vi "Handle State Value Table Change.vi"(8 "error in (no error)":errorcluster, 9 "OldVal":T1[](array[typedef]), 10 "NewVal":T1[](array[typedef]), 11 "routing channel in":T2 format="%.0x") -> (0 "error out":errorcluster, 1 "old modified state and value":T1, 2 "new modified state and value":T1, 3 "routing channel out":T2 format="%.0x", 4 "update controls":bool, 5 "coerced newval":T1[](array[typedef]))   [LabVIEW 2020, in "Routing and Faulting System Explorer.lvlib"]
uses:
  Routing and Faulting System Explorer.lvlib
  <vilib>/NI VeriStand/Custom Device API/Custom Device Item Ref.ctl
  State-Value Row.ctl
  88e8a73d-5bf6-438f-825b-ec6305f3fa8d.vi
  Scripting/Routing and Faulting Scripting.lvlib
  <vilib>/NI VeriStand/Custom Device API/Custom Device API.lvlib
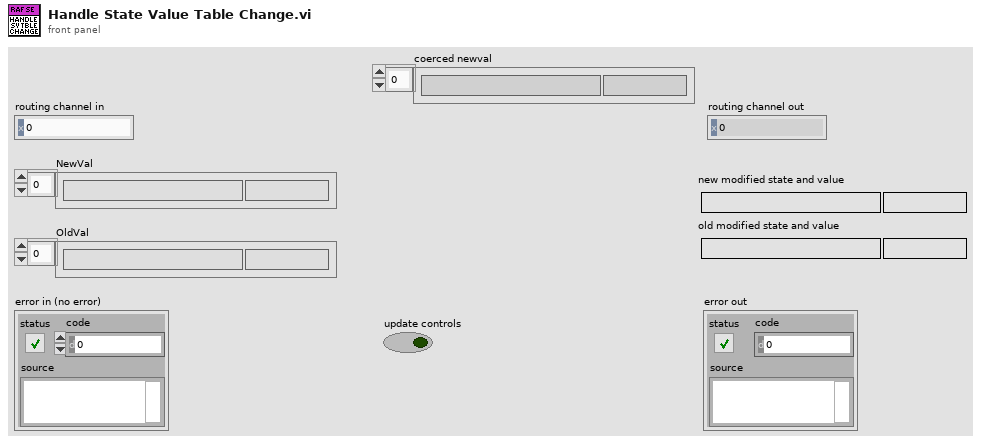
[diagram p1: front panel]
types:
  T1 = typedef "Routing and Faulting System Explorer.lvlib/State-Value Row.ctl" = cluster{"State":string, "State Value":string}
  T2 = typedef "Custom Device API.lvlib/Custom Device Item Ref.ctl" = u64
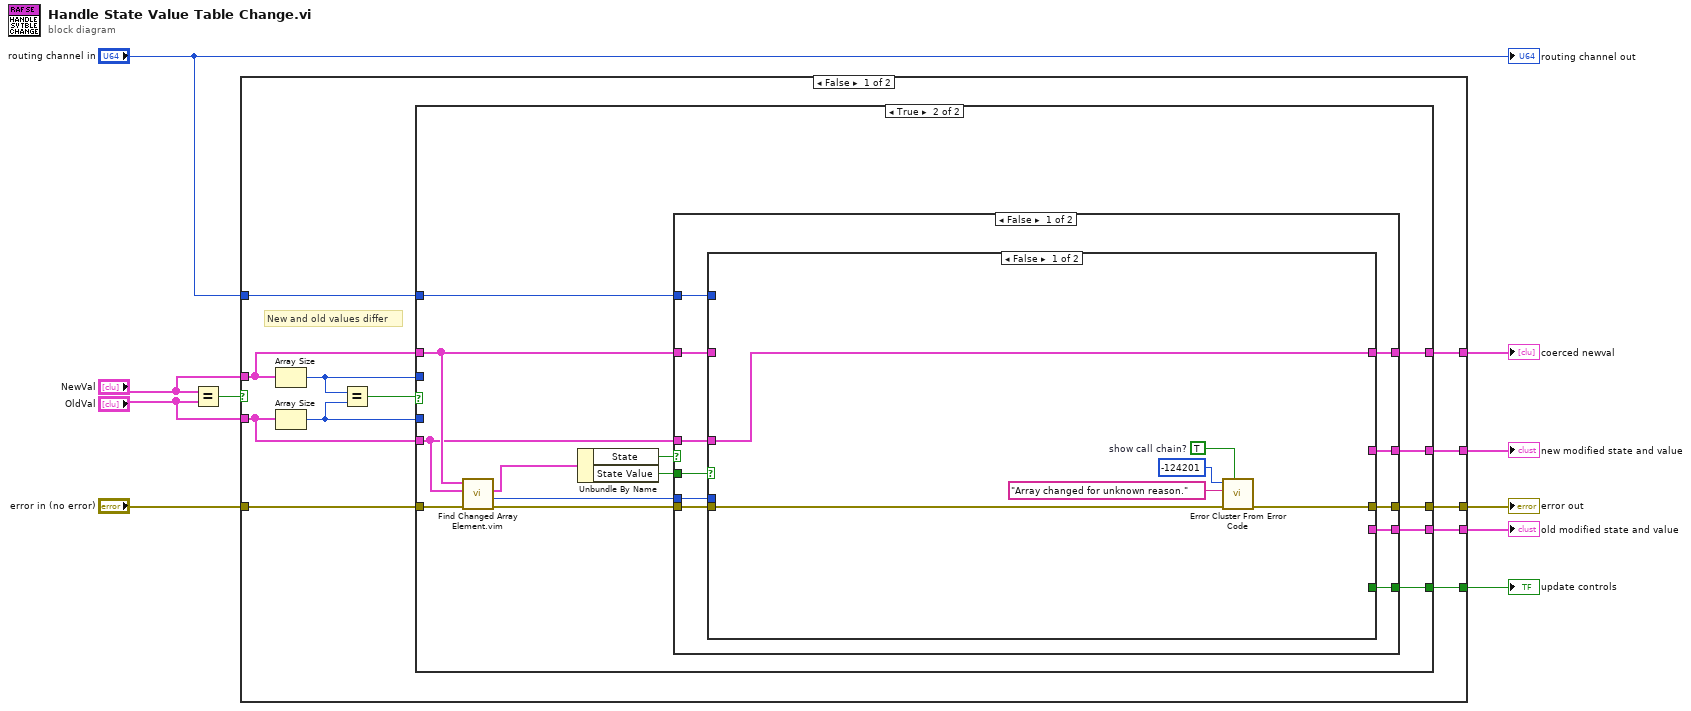
[diagram p0: block diagram]
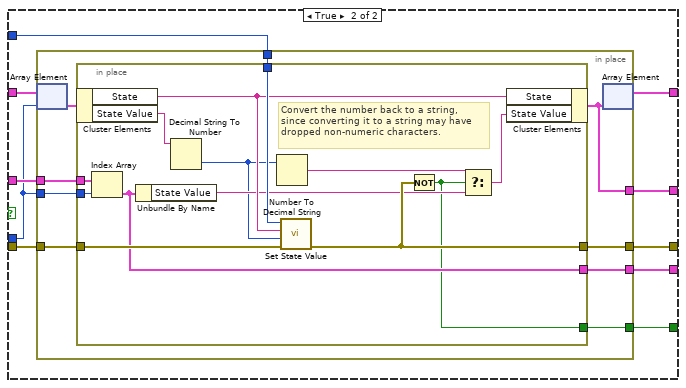
[diagram p3: hidden frame]
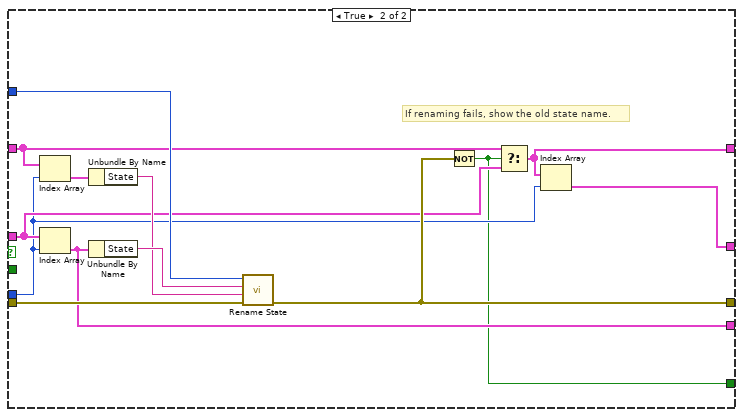
[diagram p4: hidden frame]
diagram:
  n1 = Equal?(x="NewVal", y="OldVal") -> (x = y?=w5:bool)
  n2 = case shown="False" w5 {
    tunnel: "NewVal" -> [w19 w101]
    tunnel: "OldVal" -> [w18 _]
    tunnel: "routing channel in" -> [w17 _]
    tunnel: [w16 w102] -> w10
    tunnel: "error in (no error)" -> [w15 w102]
    tunnel: [w14 w101] -> w4
    tunnel: [w13 _] -> w2
    tunnel: [w12 _] -> w1
    tunnel: [w11 _] -> w3
    frame False {
      # "New and old values differ"
      n3 = Array Size(array=w19) -> (size(s)=w21:i32)
      n4 = Array Size(array=w18) -> (size(s)=w20:i32)
      n5 = Equal?(x=w21, y=w20) -> (x = y?=w22:bool)
      n6 = case shown="True" w22 {
        tunnel: w21 -> [_ _]
        tunnel: w20 -> [_ _]
        tunnel: w19 -> [_ w34]
        tunnel: w18 -> [w23 w29]
        tunnel: w17 -> [_ w36]
        tunnel: [w24 w33] -> w16
        tunnel: w15 -> [w24 w32]
        tunnel: [w23 w30] -> w14
        tunnel: [_ w27] -> w11
        tunnel: [_ w26] -> w12
        tunnel: [_ w25] -> w13
        frame False {
          # "This case can happen if items are inserted or removed from the array\nshortcut menu during runtime. This is a lot of extra code to handle,\nso the shortcut menu for the array on Endpoint Aliases Page.vi is\ncurrently disabled to prevent this code path.\nIf the shortcut menu is ever re-enabled, code for handling add/remove\nshould go in this case."
        }
        frame True {
          n7 = call "Find Changed Array Element.vim"("error in (no error)"=w32, "OldVal"=w29, "NewVal"=w34) -> ("error out"=w35:errorcluster, "Array Index"=w28:i32, "Element Changed"=w38:cluster{"State":bool, "State Value":bool})  [unwired: 6 in]
          n8 = Unbundle By Name(w38) -> ("State"=w37:bool, "State Value"=w31:bool)
          n9 = case shown="False" w37 {
            tunnel: w36 -> [w49 w100]
            tunnel: w35 -> [w46 w99]
            tunnel: w34 -> [w45 w94]
            tunnel: w29 -> [w42 w92]
            tunnel: [w47 w95] -> w33
            tunnel: w28 -> [w44 w90]
            tunnel: w31 -> [w48 _]
            tunnel: [w43 w93] -> w30
            tunnel: [w40 w91] -> w26
            tunnel: [w41 w89] -> w27
            tunnel: [w39 w88] -> w25
            frame False {
              n10 = case shown="False" w48 {
                tunnel: w49 -> [_ w63]
                tunnel: [w55 w64] -> w47
                tunnel: w46 -> [w50 w65]
                tunnel: w45 -> [_ w62]
                tunnel: w44 -> [_ w59]
                tunnel: [w51 w61] -> w43
                tunnel: w42 -> [w51 w60]
                tunnel: [_ w58] -> w41
                tunnel: [_ w57] -> w40
                tunnel: [_ w56] -> w39
                frame False {
                  w52 = TRUE  # show call chain?
                  n11 = call <vilib>:"Error Cluster From Error Code.vi"("show call chain? (False)"=w52, "error in (no error)"=w50, "error message (\"\")"="Array changed for unknown reason." ("error message (\"\")"), "error code (0)"=-124201) -> ("error out"=w55:errorcluster)  [unwired: 5 in]
                }
                frame True {
                  n12 = in-place {
                    in-place-border: w65 -> [w74]
                    in-place-border: [w73] -> w64
                    in-place-border: w63 -> [w72]
                    in-place-border: w60 -> [w70]
                    in-place-border: w59 -> [w69]
                    in-place-border: [w68] -> w58
                    in-place-border: [w67] -> w57
                    in-place-border: [w66] -> w56
                    n13 = in-place-array #1(w62, w59) -> (w71:T1)
                    n14 = in-place {
                      in-place-border: w74 -> [w87]
                      in-place-border: [w86] -> w73
                      in-place-border: w72 -> [w85]
                      in-place-border: w70 -> [w81]
                      in-place-border: w69 -> [w80]
                      in-place-border: [w76] -> w67
                      in-place-border: [w75] -> w66
                      # "Convert the number back to a string,\nsince converting it to a string may have\ndropped non-numeric characters."
                      n15 = in-place-cluster #2(w71) -> ("State"=w82:string, "State Value"=w84:string)
                      n16 = Index Array(array=w81, index=w80) -> (element=w76:T1)
                      n17 = Unbundle By Name(w76) -> ("State Value"=w79:string)
                      n18 = Decimal String To Number(string=w84) -> (number=w78:i32)  [unwired: 2 in, 1 out]
                      n19 = Number To Decimal String(number=w78) -> (decimal integer string=w77:string)  [unwired: 1 in]
                      n20 = call "Set State Value.vi"("error in"=w87, "value"=w78, "state"=w82, "routing channel in"=w85) -> ("error out"=w86:errorcluster)  [unwired: 6 in, 1 out]
                      n21 = Not(x=w86) -> (.not. x?=w75:bool)
                      n22 = Select(t=w77, s=w75, f=w79) -> (s? t:f=w83:string)
                      n23 = in-place-cluster #2("State"=w82, "State Value"=w83) -> (w68:T1)
                    }
                    n24 = in-place-array #1(w68) -> (w61:T1[])  [unwired: 1 out]
                  }
                }
              }
            }
            frame True {
              # "If renaming fails, show the old state name."
              n25 = Index Array(array=w94, index=w90) -> (element=w98:T1)
              n26 = Index Array(array=w92, index=w90) -> (element=w91:T1)
              n27 = Unbundle By Name(w98) -> ("State"=w96:string)
              n28 = Unbundle By Name(w91) -> ("State"=w97:string)
              n29 = call "Rename State.vi"("error in"=w99, "new state"=w96, "state"=w97, "routing channel in"=w100) -> ("error out"=w95:errorcluster)  [unwired: 6 in, 1 out]
              n30 = Not(x=w95) -> (.not. x?=w88:bool)
              n31 = Select(t=w94, s=w88, f=w92) -> (s? t:f=w93:T1[])
              n32 = Index Array(array=w93, index=w90) -> (element=w89:T1)
            }
          }
        }
      }
    }
    frame True {
      # "New and old values are the same. Do nothing"
    }
  }
  "error out" <- w10
  "coerced newval" <- w4
  "new modified state and value" <- w3
  "old modified state and value" <- w1
  "update controls" <- w2
  "routing channel out" <- "routing channel in"
